vi "example test.vi"() -> ()   [LabVIEW 2014, in "UI reference module tests.lvlib"]
uses:
  UI reference module tests.lvlib
  module/configuration/UI Reference configuration old.lvclass
  module/execution/UI Reference runtime old.lvclass
  <vilib>/NI/Tag Bus/dictionary/data dictionary.lvclass
  <vilib>/NI/Tag Bus/dictionary/lookup polymorphs/locate double.vi
  <vilib>/NI/Tag Bus/table/data table.lvlib
  <vilib>/NI/Tag Bus/table/data polymorphs/write one/write Double.vi
  <vilib>/NI/Tag Bus/dictionary/lookup polymorphs/locate Boolean.vi
  <vilib>/NI/Tag Bus/dictionary/lookup polymorphs/locate String.vi
  <vilib>/NI/Tag Bus/tag/tag descriptor.lvclass
  <vilib>/NI/Tag Bus/tag/Data Type.ctl
  <vilib>/NI/Tag Bus/table/data polymorphs/write one/write Boolean.vi
  <vilib>/NI/Tag Bus/table/data polymorphs/write one/write String.vi
  <vilib>/NI/Tag Bus/table/data polymorphs/read one/read Boolean.vi
  <vilib>/NI/Tag Bus/table/data polymorphs/read one/read Double.vi
  <vilib>/NI/Tag Bus/table/data polymorphs/read one/read String.vi
  <vilib>/Analysis/NI_AALBase.lvlib
  <vilib>/Analysis/baseanly.llb/Mean (DBL).vi
  <vilib>/NI/Configuration Framework/serializable configuration/NISE_CEF_serializable configuration.lvclass
panel:
  out "out":dbl
  out "in":dbl
  out "valid times":bool
  out "u8 out":u8
  out "exec settings":errorcluster
  in  "Stop wkaround":errorcluster
  out "String out":string
  in  "String in":string
  out "bool out":bool
  in  "bool in":bool
  out "dbl out":dbl
  in  "dbl in":dbl
  out "final error":errorcluster
  out "init error":errorcluster
  out "serialization problem":errorcluster
  out "invalid configuration":errorcluster
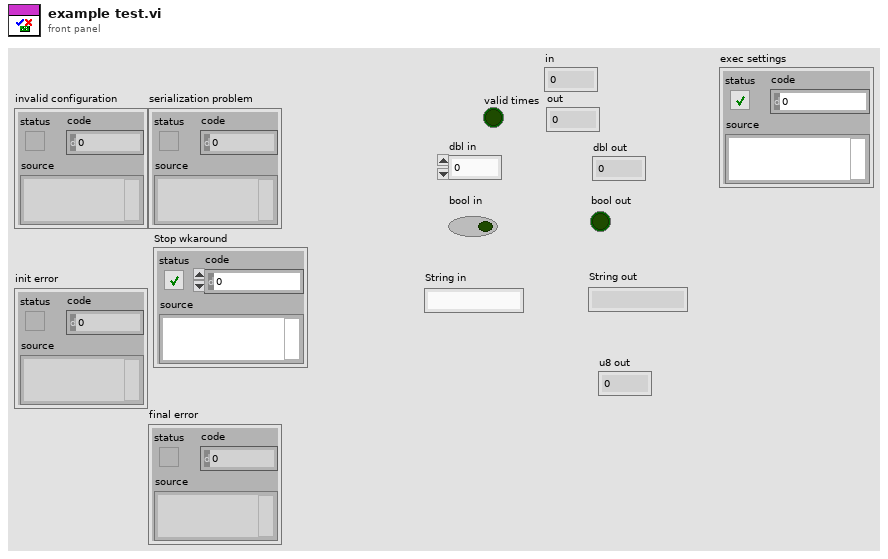
[diagram p1: front panel]
types:
  T1 = typedef "tag bus.lvlib/tag descriptor.lvclass/Data Type.ctl" = enum16{"Double", "Single", "I64", "I32", "I16", "I8", "U64", "U32", "U16", "U8", "Boolean", "String", "Array of Double", "Array of Single", "Array of I64", "Array of I32", "Array of I16", "Array of I8", "Array of U64", "Array of U32", "Array of U16", "Array of U8", "Array of Boolean", "Array of String"}
  T2 = typedef "TBM channel.lvclass/data tables.ctl" = cluster{"input data":T3, "processing parameter":T3, "processing result":T3, "output data":T3}
  T3 = typedef "tag bus.lvlib/dictionary table pair.ctl" = cluster{"data dictionary":refnum<class "data dictionary.lvclass">, "data table":T4}
  T4 = typedef "tag bus.lvlib/data table.lvlib/data table.ctl" = cluster{"Double":dbl[], "Single":sgl[], "I64":i64[], "I32":i32[], "I16":i16[], "I8":i8[], "U64":u64[], "U32":u32[], "U16":u16[], "U8":u8[], "Boolean":bool[], "String":string[], "Array of Double":cluster{"DBL Array":dbl[]}[], "Array of Single":cluster{"SGL Array":sgl[]}[], "Array of I64":cluster{"I64 Array":i64[]}[], "Array of I32":cluster{"I32 Array":i32[]}[], "Array of I16":cluster{"I16 Array":i16[]}[], "Array of I8":cluster{"I8 Array":i8[]}[], "Array of U64":cluster{"U64 Array":u64[]}[], "Array of U32":cluster{"U32 Array":u32[]}[], "Array of U16":cluster{"U16 Array":u16[]}[], "Array of U8":cluster{"U8 Array":u8[]}[], "Array of Boolean":cluster{"Boolean Array":bool[]}[], "Array of String":cluster{"String Array":string[]}[]}
  T5 = typedef "TBM module execution interface.lvclass/execution settings.ctl" = cluster{"reads inputs":bool, "processes data":bool, "writes outputs":bool}
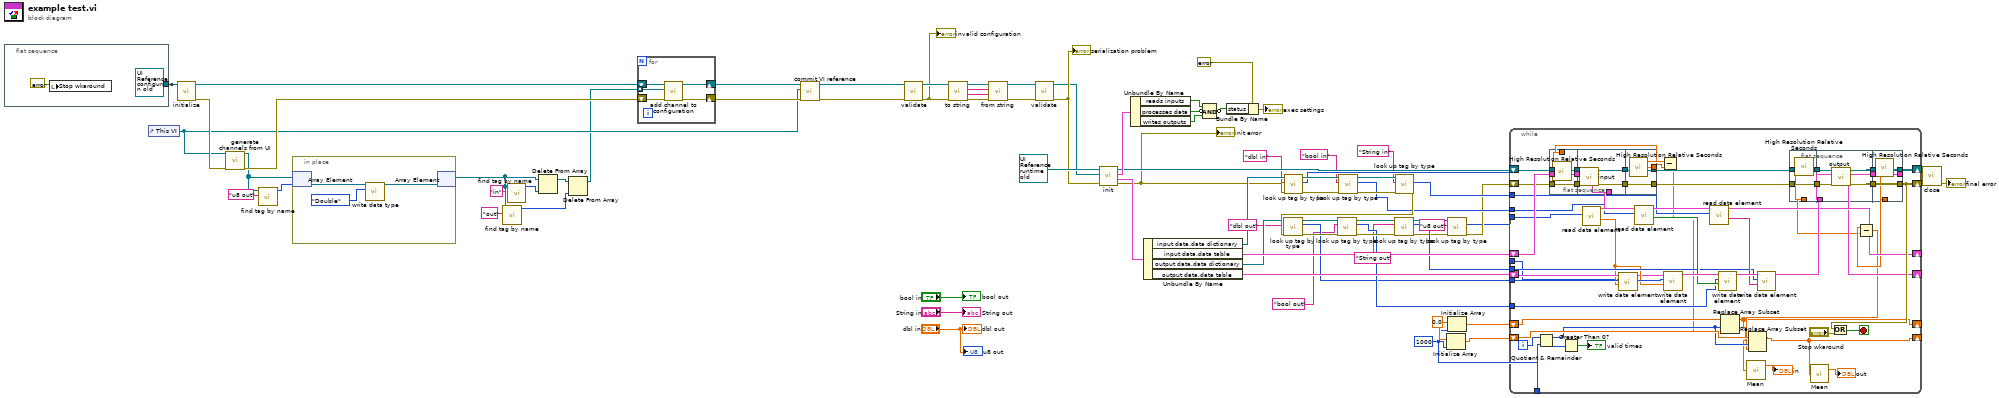
[diagram p0: block diagram]
diagram:
  w11 = 0.0 ("element")
  w8 = 1000 ("sample length")
  n1 = flat-sequence {
    tunnel: [refnum<class "UI Reference configuration old.lvclass"> refnum ("tag bus configurable plugin module configuration")] -> w60
    frame #0 {
      n2 = local write "Stop wkaround"(errorcluster {"status"=FALSE, "code"=0, "source"=""} ("Stop wkaround")) -> ()
    }
  }
  n3 = control-ref of="This VI"() -> (w12:refnum<vi>)
  n4 = call <vilib>:"initialize.vi"("configuration in"=w60) -> ("error out"=w58:errorcluster, "configuration out"=w56:refnum<class "UI Reference configuration old.lvclass">)  [unwired: 8 in, 1 out]
  n5 = call "generate channels from UI.vi"("error in"=w58, "VI Refnum"=w12) -> ("error out"=w57:errorcluster, "channels"=w22:refnum<class "TBM channel.lvclass">[])  [unwired: 8 in]
  n6 = call <vilib>:"find tag by name.vi"("name"="u8 out", "tags in"=w22) -> ("index"=w21:i32)  [unwired: 9 in]
  n7 = in-place {
    n8 = in-place-array #1(w22, w21) -> (w85:refnum<class "TBM channel.lvclass">)
    n9 = call <vilib>:"write data type.vi"("data type"=Data_Type."Double", "system tag in"=w85) -> ("system tag out"=w84:refnum<class "TBM channel.lvclass">)  [unwired: 8 in, 1 out]
    n10 = in-place-array #1(w84) -> (w5:refnum<class "TBM channel.lvclass">[])  [unwired: 1 out]
  }
  n11 = call <vilib>:"find tag by name.vi"("name"="out", "tags in"=w5) -> ("index"=w3:i32)  [unwired: 9 in]
  n12 = call <vilib>:"find tag by name.vi"("name"="in", "tags in"=w5) -> ("index"=w4:i32)  [unwired: 9 in]
  n13 = Delete From Array(array=w5, index=w4) -> (array with subset deleted=w7:refnum<class "TBM channel.lvclass">[])  [unwired: 1 in, 1 out]
  n14 = Delete From Array(array=w7, index=w3) -> (array with subset deleted=w6:refnum<class "TBM channel.lvclass">[])  [unwired: 1 in, 1 out]
  n15 = for {
    shift-right: [w90] -> w14
    shift-left: w56 -> [w88]
    shift-right: [w89] -> w59
    shift-left: w57 -> [w87]
    tunnel: w6 -> [w86] mode=indexing
    n16 = call "add channel to configuration.vi"("error in"=w87, "channel"=w86, "UI Reference configuration in"=w88) -> ("error out"=w89:errorcluster, "UI Reference configuration out"=w90:refnum<class "UI Reference configuration old.lvclass">)  [unwired: 7 in]
  }
  n17 = call "commit VI reference.vi"("error in"=w59, "VI Refnum in"=w12, "UI Reference configuration in"=w14) -> ("error out"=w15:errorcluster, "UI Reference configuration out"=w13:refnum<class "UI Reference configuration old.lvclass">)  [unwired: 6 in, 1 out]
  n18 = call-dynamic "validate.vi"("error in"=w15, "UI Reference configuration in"=w13) -> ("error out"=w79:errorcluster, "UI Reference configuration out"=w80:refnum<class "UI Reference configuration old.lvclass">)  [unwired: 8 in]
  "invalid configuration" <- w79
  n19 = call-dynamic "to string.vi"("error in"=w79, "UI Reference configuration in"=w80) -> ("error out"=w75:errorcluster, "data"=w76:string, "version"=w77:string, "UI Reference configuration out"=w78:refnum<class "UI Reference configuration old.lvclass">)  [unwired: 6 in]
  n20 = call-dynamic "from string.vi"("error in"=w75, "data"=w76, "version"=w77, "UI Reference configuration in"=w78) -> ("error out"=w73:errorcluster, "UI Reference configuration out"=w74:refnum<class "UI Reference configuration old.lvclass">)  [unwired: 6 in]
  n21 = call-dynamic "validate.vi"("error in"=w73, "UI Reference configuration in"=w74) -> ("error out"=w71:errorcluster, "UI Reference configuration out"=w70:refnum<class "UI Reference configuration old.lvclass">)  [unwired: 8 in]
  "serialization problem" <- w71
  n22 = call-dynamic "init.vi"("error in"=w71, "UI Reference configuration in"=w70, "UI Reference runtime in"=refnum<class "UI Reference runtime old.lvclass"> refnum ("tag bus configurable plugin module")) -> ("error out"=w42:errorcluster, "data allocations"=w65:T2, "execution settings"=w69:T5, "UI Reference runtime out"=w64:refnum<class "UI Reference runtime old.lvclass">)  [unwired: 5 in]
  "init error" <- w42
  n23 = Unbundle By Name(w69) -> ("reads inputs"=w66:bool, "processes data"=w68:bool, "writes outputs"=w67:bool)
  n24 = Unbundle By Name(w65) -> ("input data.data dictionary"=w43:refnum<class "data dictionary.lvclass">, "input data.data table"=w54:T4, "output data.data dictionary"=w46:refnum<class "data dictionary.lvclass">, "output data.data table"=w55:T4)
  n25 = Compound Arithmetic op=AND(w66, invert w68, w67) -> (invert w28:bool)
  n26 = Bundle By Name(cluster=errorcluster {"status"=FALSE, "code"=0, "source"=""} ("error out"), "status"=w28) -> (→"exec settings":errorcluster)
  n27 = call-poly <vilib>:"look up tag by type.vi"("error in"=w42, "name"="dbl in", "data dictionary in"=w43) -> ("error out"=w52:errorcluster, "index"=w39:i32, "data dictionary out"=w53:refnum<class "data dictionary.lvclass">)  [unwired: 6 in]
  n28 = call-poly <vilib>:"look up tag by type.vi"("error in"=w52, "name"="bool in", "data dictionary in"=w53) -> ("error out"=w50:errorcluster, "index"=w40:i32, "data dictionary out"=w51:refnum<class "data dictionary.lvclass">)  [unwired: 6 in]
  n29 = call-poly <vilib>:"look up tag by type.vi"("error in"=w50, "name"="String in", "data dictionary in"=w51) -> ("error out"=w47:errorcluster, "index"=w41:i32)  [unwired: 6 in, 1 out]
  n30 = call-poly <vilib>:"look up tag by type.vi"("error in"=w47, "name"="dbl out", "data dictionary in"=w46) -> ("error out"=w48:errorcluster, "index"=w36:i32, "data dictionary out"=w45:refnum<class "data dictionary.lvclass">)  [unwired: 6 in]
  n31 = call-poly <vilib>:"look up tag by type.vi"("error in"=w48, "name"="bool out", "data dictionary in"=w45) -> ("error out"=w49:errorcluster, "index"=w37:i32, "data dictionary out"=w44:refnum<class "data dictionary.lvclass">)  [unwired: 6 in]
  n32 = call-poly <vilib>:"look up tag by type.vi"("error in"=w49, "name"="String out", "data dictionary in"=w44) -> ("error out"=w20:errorcluster, "index"=w38:i32, "data dictionary out"=w19:refnum<class "data dictionary.lvclass">)  [unwired: 6 in]
  n33 = Initialize Array(w11, w8) -> (w9:dbl[])
  n34 = call-poly <vilib>:"look up tag by type.vi"("error in"=w20, "name"="u8 out", "data dictionary in"=w19) -> ("error out"=w18:errorcluster, "index"=w17:i32)  [unwired: 6 in, 1 out]
  n35 = Initialize Array(w11, w8) -> (w10:dbl[])
  n36 = while {
    shift-right: [w132] -> w62
    shift-left: w18 -> [w134]
    shift-right: [w143] -> w63
    shift-left: w64 -> [w146]
    tunnel: w41 -> [w129]
    tunnel: w40 -> [w128]
    tunnel: w39 -> [w127]
    tunnel: w38 -> [w126]
    tunnel: w37 -> [w125]
    tunnel: w36 -> [w124]
    tunnel: w17 -> [w121]
    shift-right: [w119] -> _
    shift-left: w54 -> [w135]
    shift-right: [w118] -> _
    shift-left: w55 -> [w123]
    shift-right: [w93] -> _
    shift-left: w10 -> [w98]
    shift-right: [w94] -> _
    shift-left: w9 -> [w99]
    tunnel: w8 -> [w102]
    i -> [w103]
    stop <- w130 stop-if-true
    n37 = Quotient & Remainder(x=w103, y=w102) -> (x-y*floor(x/y)=w97:i32, floor(x/y)=w101:i32)
    n38 = flat-sequence {
      tunnel: w134 -> [w161]
      tunnel: w135 -> [w162]
      tunnel: w146 -> [w163]
      tunnel: [w163] -> w115
      tunnel: [w162] -> w114
      tunnel: [w161] -> w113
      tunnel: [w160] -> w106
      tunnel: [w164] -> w133
      tunnel: [w168] -> w117
      tunnel: [w167] -> w116
      tunnel: w115 -> [w169]
      tunnel: w114 -> [w166]
      tunnel: w113 -> [w165]
      tunnel: [w171] -> w142
      tunnel: [w172] -> w145
      tunnel: w117 -> [w172]
      tunnel: w116 -> [w171]
      tunnel: [w170] -> w107
      frame #0 {
        n39 = call <vilib>:"High Resolution Relative Seconds.vi"() -> ("relative seconds"=w160:dbl)
      }
      frame #1 {
        n40 = call-dynamic "input.vi"("error in"=w165, "data table in"=w166, "UI Reference runtime in"=w169) -> ("error out"=w167:errorcluster, "data table out"=w164:T4, "UI Reference runtime out"=w168:refnum<class "UI Reference runtime old.lvclass">)  [unwired: 6 in]
      }
      frame #2 {
        n41 = call <vilib>:"High Resolution Relative Seconds.vi"() -> ("relative seconds"=w170:dbl)
      }
    }
    n42 = Greater Than 0?(x=w101) -> (x > 0?=→"valid times":bool)
    n43 = call-poly <vilib>:"read data element.vi"("index"=w127, "data table in"=w133) -> ("value"=w122:dbl, "data table out"=w139:T4)  [unwired: 8 in]
    n44 = call-poly <vilib>:"write data element.vi"("value"=w122, "index"=w121, "data table in"=w123) -> ("data table out"=w120:T4)  [unwired: 8 in]
    n45 = call-poly <vilib>:"read data element.vi"("index"=w128, "data table in"=w139) -> ("value"=w136:bool, "data table out"=w138:T4)  [unwired: 8 in]
    n46 = Subtract(x=w107, y=w106) -> (x-y=w96:dbl)
    n47 = call-poly <vilib>:"write data element.vi"("value"=w122, "index"=w124, "data table in"=w120) -> ("data table out"=w140:T4)  [unwired: 8 in]
    n48 = call-poly <vilib>:"read data element.vi"("index"=w129, "data table in"=w138) -> ("value"=w137:string, "data table out"=w119:T4)  [unwired: 8 in]
    n49 = call-poly <vilib>:"write data element.vi"("value"=w136, "index"=w125, "data table in"=w140) -> ("data table out"=w141:T4)  [unwired: 8 in]
    n50 = Replace Array Subset(array=w98, new element=w96, index=w97) -> (w93:dbl[])
    n51 = call-poly <vilib>:"Mean.vi"("X"=w93) -> ("mean"=→"in":dbl)  [unwired: 1 out]
    n52 = call-poly <vilib>:"write data element.vi"("value"=w137, "index"=w126, "data table in"=w141) -> ("data table out"=w144:T4)  [unwired: 8 in]
    n53 = flat-sequence {
      tunnel: w142 -> [w148]
      tunnel: w145 -> [w149]
      tunnel: [w149] -> w109
      tunnel: [w148] -> w108
      tunnel: [w147] -> w104
      tunnel: w144 -> [w154]
      tunnel: [w153] -> w112
      tunnel: [w151] -> w111
      tunnel: [w150] -> w110
      tunnel: w109 -> [w155]
      tunnel: w108 -> [w152]
      tunnel: [w157] -> w118
      tunnel: [w158] -> w132
      tunnel: [w159] -> w143
      tunnel: w112 -> [w159]
      tunnel: w111 -> [w158]
      tunnel: w110 -> [w157]
      tunnel: [w156] -> w105
      frame #0 {
        n54 = call <vilib>:"High Resolution Relative Seconds.vi"() -> ("relative seconds"=w147:dbl)
      }
      frame #1 {
        n55 = call-dynamic "output.vi"("error in"=w152, "data table in"=w154, "UI Reference runtime in"=w155) -> ("error out"=w151:errorcluster, "data table out"=w150:T4, "UI Reference runtime out"=w153:refnum<class "UI Reference runtime old.lvclass">)  [unwired: 6 in]
      }
      frame #2 {
        n56 = call <vilib>:"High Resolution Relative Seconds.vi"() -> ("relative seconds"=w156:dbl)
      }
    }
    n57 = Or(x=w132, y="Stop wkaround") -> (x .or. y?=w130:bool)
    n58 = Subtract(x=w105, y=w104) -> (x-y=w95:dbl)
    n59 = Replace Array Subset(array=w99, new element=w95, index=w97) -> (w94:dbl[])
    n60 = call-poly <vilib>:"Mean.vi"("X"=w94) -> ("mean"=→"out":dbl)  [unwired: 1 out]
  }
  n61 = call-dynamic "close.vi"("error in"=w62, "UI Reference runtime in"=w63) -> ("error out"=→"final error":errorcluster)  [unwired: 9 in]
  "dbl out" <- "dbl in"
  "bool out" <- "bool in"
  "String out" <- "String in"
  "u8 out" <- "dbl in"
